vi "Horizontal Range Increment.vi"(7 "steps":i32(ring) caption="Steps" items=["ZTSCOPEM_INCREMENT", "ZTSCOPEM_DECREMENT"], 8 "error in":errorcluster, 10 "Nominal Points":u32, 11 "Instrument Handle In":i32) -> (0 "error out":errorcluster, 1 "Interpolating":i32, 2 "Actual Nominal Points":u32, 3 "Instrument Handle Out":i32)   [LabVIEW 8.6, in "ZTScopeM.lvlib"]
doc: "Increment the instrument's horizontal time and point settings to acquire the next possible sample rate.\n\nExample:\nIf the current instrument settings are:\n1 MS/s with 1000 points = 1 ms\n\nPassing in steps=\"Up\" with Nominal Points = 1000 will change the settings to:\n2 MS/s with 1000 points = 500 us\nActual Nominal Points = 1000, Interpolating = 0\n\nIf the maximum real-time sample rate of the instrument is 1MS/s, the same request would set:\n1 MS/s with 500 points = 500 us\nActual Nominal Points = 1000, Interpolating = 1\nThese settings still result in an interpolated rate of 2 MS/s when 1000 points are downloaded over the timespan.\n\nActual Nominal Points is coerced if the new sample rate is not achievable with the requested Nominal Points, Using the example above, if the user requested steps=\"Up\" with Nominal Points = 10, the function would normally attempt to set \n1 MS/s with 5 points = 50 us, Nominal Points = 10\nActual Nominal Points = 10, Interpolating = 1\n\nHowever, the instrument cannot capture less than 10 points. Instead the settings would become:\n1 MS/s with 10 points = 100 us\nActual Nominal Points = 20, Interpolating = 1\n\nThis coercion of the nominal points may also occur if the resulting rate would require a non-integer interpolation"
uses:
  ZTScopeM.lvlib
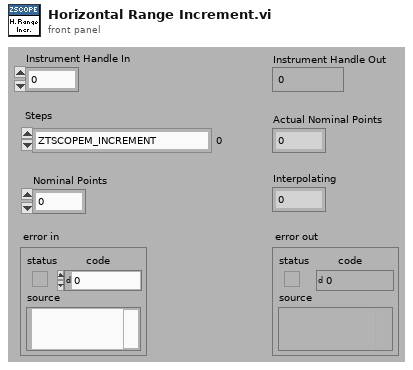
[diagram p1: front panel]
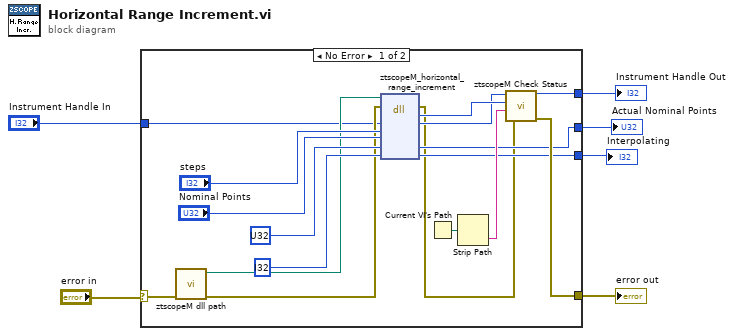
[diagram p0: block diagram]
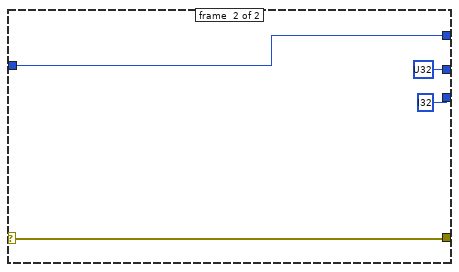
[diagram p2: hidden frame]
diagram:
  n1 = case shown="No Error" "error in" {
    selector: "error in" -> [w11 w27]
    tunnel: [w18 w27] -> w5
    tunnel: [w19 w24] -> w4
    tunnel: [w15 i32 ? ("interpolating")] -> w3
    tunnel: [w13 u32 ? ("actualNominalPoints")] -> w2
    tunnel: "Instrument Handle In" -> [w7 w24]
    frame #0 {
      n2 = call "ztscopeM dll path.vi"("error in (no error)"=w11) -> ("error out"=w9:errorcluster, "<instrument>.dll path"=w10:path)  [unwired: 9 in]
      n3 = dll-call lib="C:/Program Files (x86)/National Instruments/LabVIEW 2013/instr.lib/ztscopem/ztscopeM.dll" fn="ztscopeM_horizontal_range_increment"(path in=w10, error in=w9, "instrumentHandle"=w7, "steps"="steps", "nominalPoints"="Nominal Points", "actualNominalPoints"=u32 ?, "interpolating"=i32 ?) -> (error out=w8:errorcluster, w23:i32, "instrumentHandle"=w22:i32, "actualNominalPoints"=w13:u32, "interpolating"=w15:i32)  [unwired: 3 in, 1 out]
      n4 = Current VI's Path() -> (path=w21:path)
      n5 = Strip Path(path=w21) -> (name=w20:string)  [unwired: 1 out]
      n6 = call "ztscopeM Check Status.vi"("error in"=w8, "name of VI"=w20, "status (return code)"=w23, "instrument handle in"=w22) -> ("error out"=w18:errorcluster, "instrument handle out"=w19:i32)  [unwired: 2 out]
    }
    frame #1 {
    }
  }
  "Instrument Handle Out" <- w4
  "error out" <- w5
  "Interpolating" <- w3
  "Actual Nominal Points" <- w2
